vi "get_value.vi"(8 "error in (no error)":errorcluster, 11 "Dimension in":refnum<class "Dimension.lvclass">) -> (0 "error out":errorcluster, 1 "is_set?":bool, 2 "value":T1, 3 "Dimension out":refnum<class "Dimension.lvclass">)   [LabVIEW 2020, in "mlir.lvlib" / "Dimension.lvclass"]
uses:
  Dimension.lvclass
  Dimension.lvclass/Dimension.ctl
  value.ctl
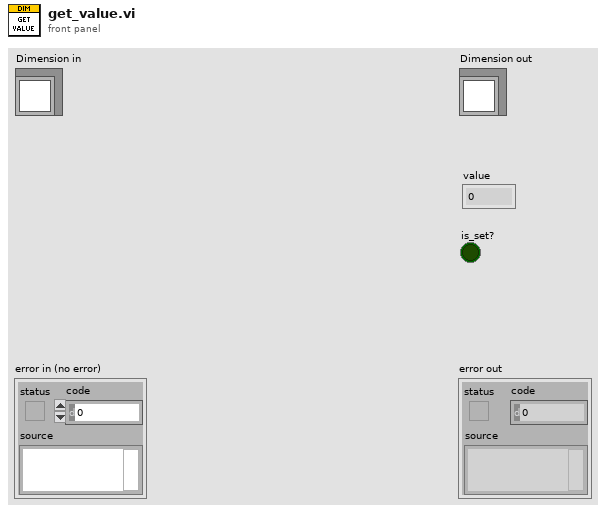
[diagram p1: front panel]
types:
  T1 = typedef "mlir.lvlib/Dimension.lvclass/value.ctl" = u32
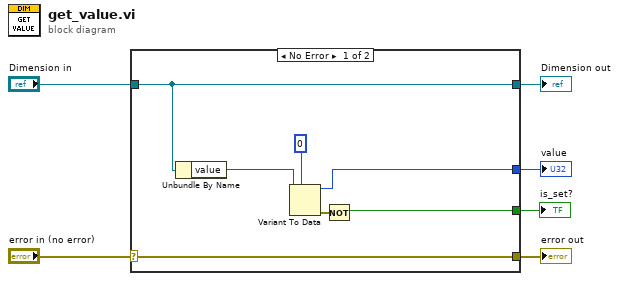
[diagram p0: block diagram]
diagram:
  n1 = case shown="No Error" "error in (no error)" {
    selector: "error in (no error)" -> [w13 w14]
    tunnel: [w13 w14] -> w5
    tunnel: [w12 w15] -> w3
    tunnel: "Dimension in" -> [w12 w15]
    tunnel: [w8 _] -> w2
    tunnel: [w7 _] -> w1
    frame No Error {
      n2 = Unbundle By Name(w12) -> ("value"=w9:variant)
      n3 = Variant To Data(type=T1 0 ("value"), Variant=w9) -> (data=w8:T1, error out=w11:errorcluster)  [unwired: 1 in]
      n4 = Not(x=w11) -> (.not. x?=w7:bool)
    }
    frame Error {
    }
  }
  "error out" <- w5
  "Dimension out" <- w3
  "value" <- w2
  "is_set?" <- w1
